vi "BK Precision 913XX Output DC Volts CONTINOUS.vi"() -> ()   [LabVIEW 2017]
doc: "This example shows how to configure the instrument's output voltage level and over voltage protection. The actual voltage level and actual current level are returned."
uses:
  <instrlib>/BK Precision 913XX/BK Precision 913XX.lvlib
panel:
  in  "Voltage Level (0.0 V)":dbl format="%.3g"
  out "Actual Power Level (W)":dbl format="%.4g"
  out "Actual Voltage Level (V)":dbl format="%.4g"
  out "Actual Current Level (A)":dbl format="%.4g"
  in  "Voltage Limit (36.000 V)":dbl=36.0 min=0.0 max=66.0 step=0.001 format="%.3g"
  in  "Enable OVP (T: Enable)":bool=TRUE
  in  "Channel (1:1)":u16(ring)=1 items=["1"=1, "2"=2, "3"=3]
  in  "Current Limit (0.0 A)":dbl min=0.0 max=25.0 step=1.0 format="%.3f"
  in  "Stop Output":bool
  in  "VISA resource name":refnum<visa-resource-name>
  # "(c) 2015 B&K Precision Corporation.  ALL RIGHTS RESERVED."
  # "V"
  # "Over Voltage Protection"
  # "V"
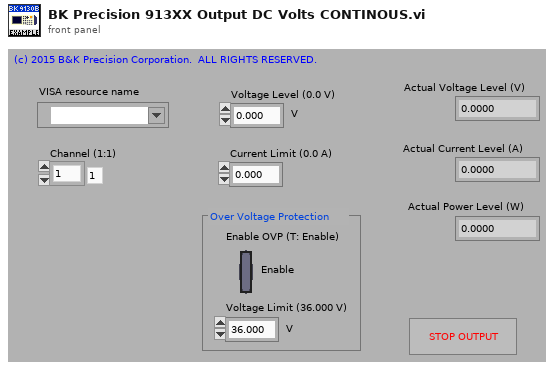
[diagram p1: front panel]
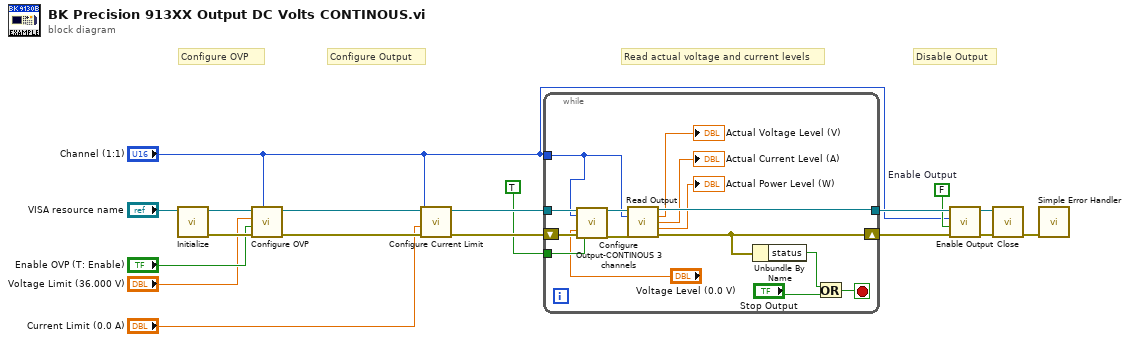
[diagram p0: block diagram]
diagram:
  w4 = FALSE  # Enable Output
  # "Disable Output"
  # "Read actual voltage and current levels"
  # "Configure Output"
  # "Configure OVP"
  n1 = call <instrlib>:"Initialize.vi"("VISA resource name"="VISA resource name") -> ("error out"=w16:errorcluster, "VISA resource name out"=w15:refnum<visa-resource-name>)  [unwired: 9 in]
  n2 = call <instrlib>:"Configure OVP.vi"("Channel (1:1)"="Channel (1:1)", "error in (no error)"=w16, "Enable OVP (T: Enable)"="Enable OVP (T: Enable)", "Voltage Limit (36.000 V)"="Voltage Limit (36.000 V)", "VISA resource name"=w15) -> ("error out"=w13:errorcluster, "VISA resource name out"=w14:refnum<visa-resource-name>)  [unwired: 5 in]
  n3 = call <instrlib>:"Configure Current Limit.vi"("error in (no error)"=w13, "Current Limit (0.0 A)"="Current Limit (0.0 A)", "Channel (1:1)"="Channel (1:1)", "VISA resource name"=w14) -> ("error out"=w9:errorcluster, "VISA resource name out"=w8:refnum<visa-resource-name>)  [unwired: 6 in]
  n4 = while {
    tunnel: w8 -> [w25]
    tunnel: [w29] -> w12
    shift-right: [w30] -> w7
    shift-left: w9 -> [w24]
    tunnel: "Channel (1:1)" -> [w19]
    tunnel: TRUE -> [w21]
    stop <- w33 stop-if-true
    n5 = call <instrlib>:"Configure Output-CONTINOUS 3 channels.vi"("VISA resource name"=w25, "Channel (1:1)"=w19, "Voltage Level (0.0 V)"="Voltage Level (0.0 V)", "error in (no error)"=w24, "Enable Channel Output (F: False)"=w21) -> ("VISA resource name out"=w22:refnum<visa-resource-name>, "error out"=w23:errorcluster)  [unwired: 13 in]
    n6 = call <instrlib>:"Read Output.vi"("VISA resource name"=w22, "Channel (1:Channel 1)"=w19, "error in (no error)"=w23) -> ("VISA resource name out"=w29:refnum<visa-resource-name>, "Actual Voltage Level (V)"=→"Actual Voltage Level (V)":dbl, "Actual Current Level (A)"=→"Actual Current Level (A)":dbl, "Actual Power Level (W)"=→"Actual Power Level (W)":dbl, "error out"=w30:errorcluster)  [unwired: 8 in]
    n7 = Unbundle By Name(w30) -> ("status"=w31:bool)
    n8 = Or(x=w31, y="Stop Output") -> (x .or. y?=w33:bool)
  }
  n9 = call <instrlib>:"Enable Output.vi"("error in (no error)"=w7, "Enable Output (F: False)"=w4, "Channel (1:1)"="Channel (1:1)", "VISA resource name"=w12) -> ("error out"=w10:errorcluster, "VISA resource name out"=w11:refnum<visa-resource-name>)  [unwired: 6 in]
  n10 = call <instrlib>:"Close.vi"("error in (no error)"=w10, "VISA resource name"=w11) -> ("error out"=w17:errorcluster)  [unwired: 9 in]
  n11 = call <vilib>:"Simple Error Handler.vi"("error in (no error)"=w17) -> ()  [unwired: 4 in, 5 out]
